vi "g2_2D.vi"() -> ()   [LabVIEW 2020]
uses:
  <vilib>/Math Plots/2D Math Plots/2D Error Bar/2D Error Bar XCtrl/2D Error Bar.xctl
  C:/Program Files/Dotfast Consulting/Timetag Explorer 2.26/ttInterface.dll
  Program Files/Dotfast Consulting/Timetag Explorer 2.26/ttInterface.dll
  <vilib>/Utility/file.llb/Write Delimited Spreadsheet (I64).vi
  <vilib>/Math Plots/2D Math Plots/2D Error Bar/2D Error Bar Datatype/Public/Plot Helper (Fixed).vi
  <vilib>/Math Plots/2D Math Plots/2D Error Bar/2D Error Bar Datatype/2D Error Bar Datatype.lvclass
  <vilib>/Analysis/NI_AALBase.lvlib
panel:
  out "Intensity Graph":dbl[][](graph)
  out "Numeric 2":i32
  out "Current Delay":dbl
  out "appended array":i32[](array[numeric])
  out "ABC":refnum<class "2D Plot Datatype.lvclass">[](xcontrol)
  out "Numeric":i32
  in  "Acq Time (s)":dbl=0.1 format="%#_13g"
  out "BC":refnum<class "2D Plot Datatype.lvclass">[](xcontrol)
  in  "# Steps":i32
  in  "stop":bool
  in  "fileName":string
  in  "Folder":path
  in  "CTW in ns":dbl
  out "GetTimeCounter":i32
  out "GetResolution":dbl
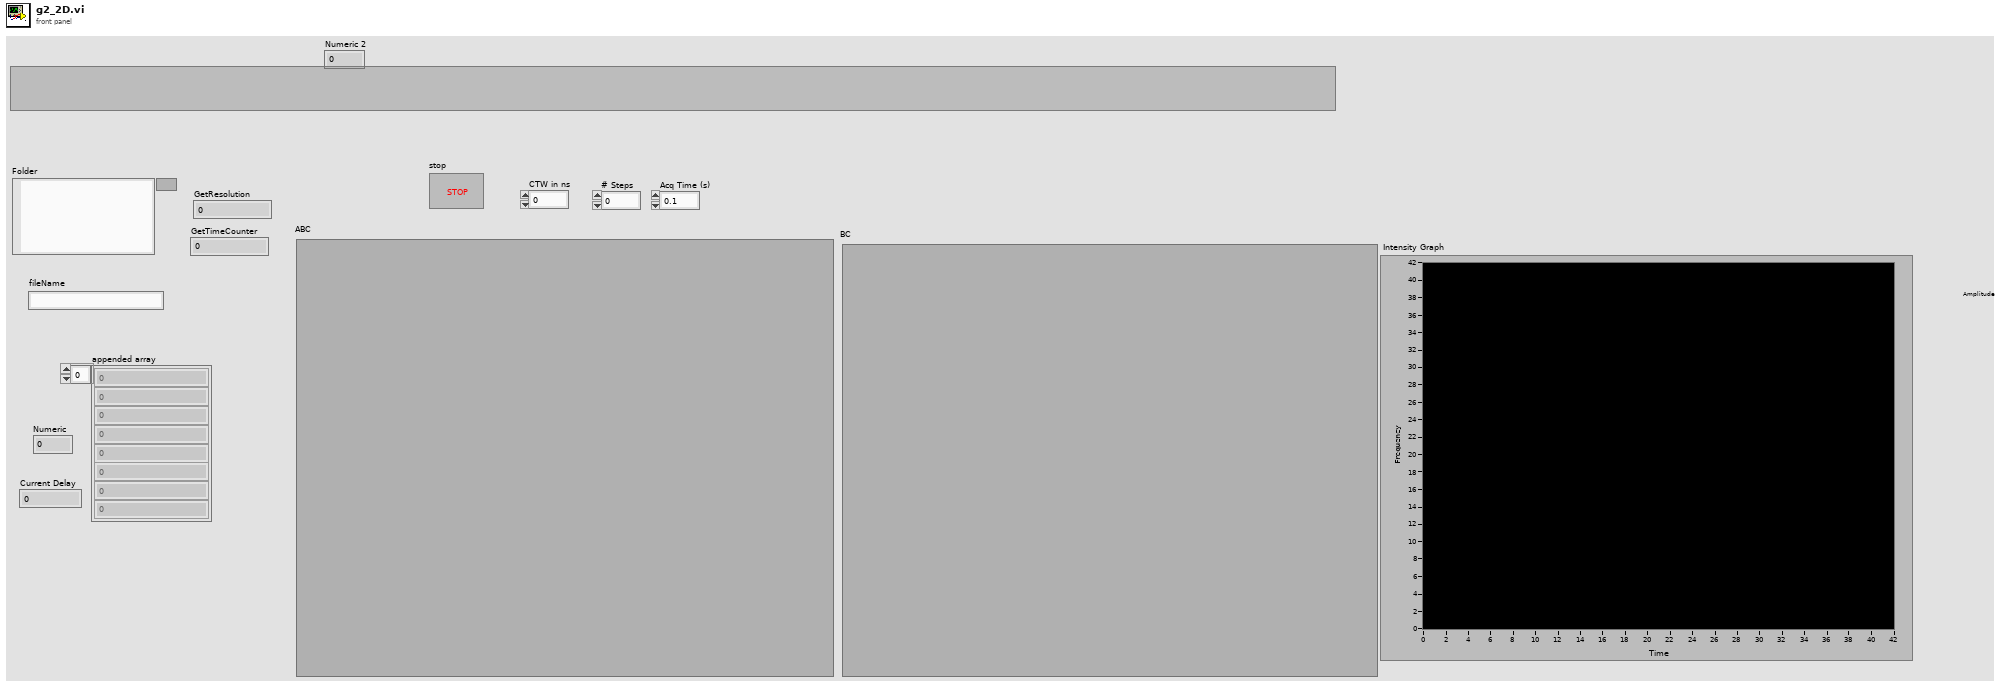
[diagram p1: front panel]
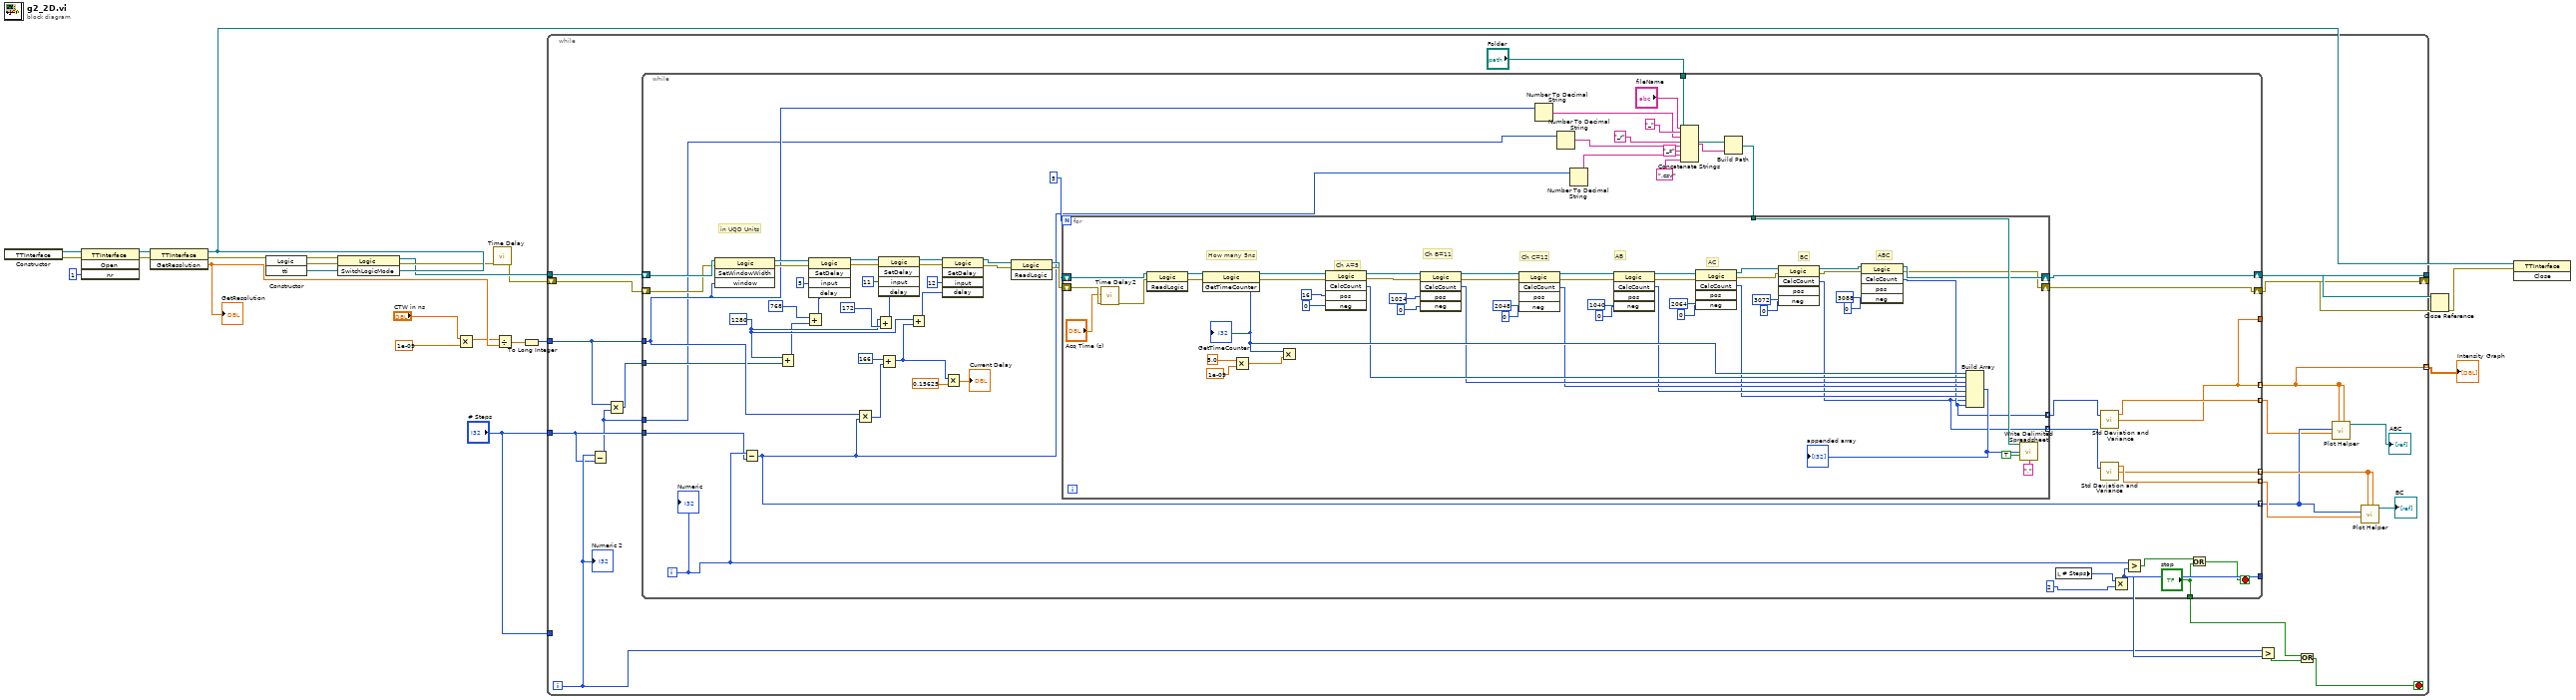
[diagram p0: block diagram]
diagram:
  n1 = constructor class="TTInterface"() -> (reference out=w23:refnum<k24>, error out=w22:errorcluster)  [unwired: 3 in, 1 out]
  n2 = invoke class="TTInterface" method="Open"(reference=w23, error in=w22, "nr"=1) -> (reference out=w19:refnum<k24>, error out=w20:errorcluster)  [unwired: 1 in, 2 out]
  n3 = invoke class="TTInterface" method="GetResolution"(reference=w19, error in=w20) -> (reference out=w18:refnum<k24>, error out=w17:errorcluster, "GetResolution"=w11:dbl)  [unwired: 1 in]
  "GetResolution" <- w11
  n4 = constructor class="Logic"(error in=w17, "tti"=w18) -> (reference out=w16:refnum<k24>, error out=w15:errorcluster)  [unwired: 2 in, 2 out]
  n5 = invoke class="Logic" method="SwitchLogicMode"(reference=w16, error in=w15) -> (reference out=w13:refnum<k24>, error out=w14:errorcluster)  [unwired: 1 in, 1 out]
  n6 = Multiply(x="CTW in ns", y=1e-09) -> (x*y=w10:dbl)
  n7 = call "Time Delay"("error in (no error)"=w14) -> ("error out"=w12:errorcluster)  [unwired: 10 in]
  n8 = Divide(x=w10, y=w11) -> (x/y=w9:dbl)
  n9 = To Long Integer(number=w9) -> (32bit integer=w6:i32)
  n10 = while {
    tunnel: w13 -> [w44]
    tunnel: w6 -> [w27]
    tunnel: "# Steps" -> [w28]
    shift-right: [w40] -> w3
    shift-left: w12 -> [w43]
    tunnel: [w41] -> w5
    tunnel: "# Steps" -> [_]
    tunnel: [w24] -> w1 mode=indexing
    i -> [w29]
    stop <- w30 stop-if-true
    n11 = Subtract(x=w29, y=w28) -> (x-y=w25:i32)
    n12 = Multiply(x=w27, y=w25) -> (x*y=w26:i32)
    n13 = while {
      shift-right: [w75] -> w41
      shift-left: w44 -> [w100]
      shift-right: [w74] -> w40
      shift-left: w43 -> [w99]
      tunnel: "Folder" -> [w94]
      tunnel: w27 -> [w81]
      tunnel: w28 -> [w78]
      tunnel: [w72] -> w34 mode=indexing
      tunnel: [w45] -> w24 mode=indexing
      tunnel: [w49] -> w35 mode=indexing
      tunnel: [w70] -> w36 mode=indexing
      tunnel: [w69] -> w37 mode=indexing
      tunnel: ["stop"] -> w33
      tunnel: [w53] -> w31
      tunnel: w26 -> [w47]
      tunnel: w25 -> [w46]
      tunnel: [w45] -> _
      i -> [w79]
      stop <- w91 stop-if-true
      w55 = 1280
      # "in UQD Units"
      n14 = invoke class="Logic" method="SetWindowWidth"(reference=w100, error in=w99, "window"=w81) -> (reference out=w98:refnum<k24>, error out=w97:errorcluster)  [unwired: 1 in, 2 out]
      n15 = Subtract(x=w79, y=w78) -> (x-y=w49:i32)
      n16 = Add(x=w55, y=w47) -> (x+y=w48:i32)
      n17 = Add(x=768 ("delay"), y=w48) -> (x+y=w59:i32)
      n18 = invoke class="Logic" method="SetDelay"(reference=w98, error in=w97, "input"=5, "delay"=w59) -> (reference out=w96:refnum<k24>, error out=w95:errorcluster)  [unwired: 1 in, 3 out]
      n19 = Multiply(x=w81, y=w49) -> (x*y=w80:i32)
      n20 = Add(x=w55, y=172 ("delay")) -> (x+y=w57:i32)
      n21 = invoke class="Logic" method="SetDelay"(reference=w96, error in=w95, "input"=11, "delay"=w57) -> (reference out=w89:refnum<k24>, error out=w88:errorcluster)  [unwired: 1 in, 3 out]
      n22 = Add(x=166 ("delay"), y=w80) -> (x+y=w62:i32)
      n23 = Add(x=w55, y=w62) -> (x+y=w56:i32)
      n24 = invoke class="Logic" method="SetDelay"(reference=w89, error in=w88, "input"=12, "delay"=w56) -> (reference out=w87:refnum<k24>, error out=w86:errorcluster)  [unwired: 1 in, 3 out]
      n25 = Multiply(x=w62, y=0.15625) -> (x*y=→"Current Delay":dbl)
      n26 = invoke class="Logic" method="ReadLogic"(reference=w87, error in=w86) -> (reference out=w102:refnum<k24>, error out=w103:errorcluster)  [unwired: 1 in, 1 out]
      n27 = Number To Decimal String(number=w81) -> (decimal integer string=w66:string)  [unwired: 1 in]
      n28 = Number To Decimal String(number=w46) -> (decimal integer string=w64:string)  [unwired: 1 in]
      n29 = Number To Decimal String(number=w49) -> (decimal integer string=w51:string)  [unwired: 1 in]
      n30 = Concatenate Strings("fileName", "_" ("string"), w66, "_r" ("string"), w64, "_s" ("string"), w51, ".csv" ("string")) -> (w92:string)
      n31 = Build Path(base path=w94, name or relative path=w92) -> (appended path=w93:path)
      n32 = for {
        N: 5 -> [_]
        shift-right: [w113] -> w74
        shift-left: w103 -> [w154]
        shift-right: [w114] -> w75
        shift-left: w102 -> [w153]
        tunnel: w93 -> [w140]
        tunnel: [w105] -> w73 mode=indexing
        tunnel: [w104] -> w71 mode=indexing
        # "ABC"
        # "BC"
        # "AC"
        # "AB"
        # "Ch C=12"
        # "Ch B=11"
        # "Ch A=5"
        # "How many 5ns"
        n33 = call "Time Delay2"("error in (no error)"=w154, "Delay Time (s)"="Acq Time (s)") -> ("error out"=w152:errorcluster)  [unwired: 9 in]
        n34 = invoke class="Logic" method="ReadLogic"(reference=w153, error in=w152) -> (reference out=w147:refnum<k24>, error out=w146:errorcluster)  [unwired: 1 in, 1 out]
        n35 = invoke class="Logic" method="GetTimeCounter"(reference=w147, error in=w146) -> (reference out=w144:refnum<k24>, error out=w143:errorcluster, "GetTimeCounter"=w112:i32)  [unwired: 1 in]
        "GetTimeCounter" <- w112
        n36 = Multiply(x=5.0, y=1e-09) -> (x*y=w148:dbl)
        n37 = Multiply(x=w112, y=w148) -> ()  [unwired: 1 out]
        n38 = invoke class="Logic" method="CalcCount"(reference=w144, error in=w143, "pos"=16, "neg"=0) -> (reference out=w136:refnum<k24>, error out=w135:errorcluster, "CalcCount"=w111:i32)  [unwired: 1 in, 2 out]
        n39 = invoke class="Logic" method="CalcCount"(reference=w136, error in=w135, "pos"=1024, "neg"=0) -> (reference out=w132:refnum<k24>, error out=w131:errorcluster, "CalcCount"=w110:i32)  [unwired: 1 in, 2 out]
        n40 = invoke class="Logic" method="CalcCount"(reference=w132, error in=w131, "pos"=2048, "neg"=0) -> (reference out=w128:refnum<k24>, error out=w127:errorcluster, "CalcCount"=w109:i32)  [unwired: 1 in, 2 out]
        n41 = invoke class="Logic" method="CalcCount"(reference=w128, error in=w127, "pos"=1040, "neg"=0) -> (reference out=w124:refnum<k24>, error out=w123:errorcluster, "CalcCount"=w108:i32)  [unwired: 1 in, 2 out]
        n42 = invoke class="Logic" method="CalcCount"(reference=w124, error in=w123, "pos"=2064, "neg"=0) -> (reference out=w119:refnum<k24>, error out=w120:errorcluster, "CalcCount"=w107:i32)  [unwired: 1 in, 2 out]
        n43 = invoke class="Logic" method="CalcCount"(reference=w119, error in=w120, "pos"=3072, "neg"=0) -> (reference out=w116:refnum<k24>, error out=w115:errorcluster, "CalcCount"=w104:i32)  [unwired: 1 in, 2 out]
        n44 = invoke class="Logic" method="CalcCount"(reference=w116, error in=w115, "pos"=3088, "neg"=0) -> (reference out=w114:refnum<k24>, error out=w113:errorcluster, "CalcCount"=w105:i32)  [unwired: 1 in, 2 out]
        n45 = Build Array(w112, w111, w110, w109, w108, w107, w104, w105) -> (w106:i32[])
        "appended array" <- w106
        n46 = call-poly <vilib>:"Write Delimited Spreadsheet.vi"("file path (dialog if empty)"=w140, "1D data"=w106, "append to file? (new file:F)"=TRUE, "delimiter (\\t)"="," ("delimiter (\\t)")) -> ()  [unwired: 10 in, 2 out]
      }
      n47 = local read "# Steps"() -> (w77:i32)
      n48 = call <vilib>:"Std Deviation and Variance.vi"("X"=w73) -> ("mean"=w72:dbl, "standard deviation"=w45:dbl)  [unwired: 1 in, 1 out]
      n49 = call <vilib>:"Std Deviation and Variance.vi"("X"=w71) -> ("mean"=w70:dbl, "standard deviation"=w69:dbl)  [unwired: 1 in, 1 out]
      n50 = Multiply(x=w77, y=2) -> (x*y=w53:i32)
      n51 = Greater?(x=w79, y=w53) -> (0:w90:bool)
      n52 = Or(x=w90, y="stop") -> (x .or. y?=w91:bool)
      "Numeric" <- w79
    }
    n53 = Greater?(x=w29, y=w31) -> (0:w32:bool)
    n54 = Or(x=w33, y=w32) -> (x .or. y?=w30:bool)
    n55 = call-poly <vilib>:"Plot Helper.vi"("error b vector"=w24, "error a vector"=w24, "y vector"=w34, "x vector"=w35) -> ("2D Plot Class Obj Array out"=→"ABC":refnum<class "2D Plot Datatype.lvclass">[])  [unwired: 2 in, 5 out]
    n56 = call-poly <vilib>:"Plot Helper.vi"("error b vector"=w37, "error a vector"=w37, "y vector"=w36, "x vector"=w35) -> ("2D Plot Class Obj Array out"=→"BC":refnum<class "2D Plot Datatype.lvclass">[])  [unwired: 2 in, 5 out]
    "Numeric 2" <- w29
  }
  "Intensity Graph" <- w1
  n57 = Close Reference(reference=w5, error in (no error)=w3) -> (error out=w4:errorcluster)
  n58 = invoke class="TTInterface" method="Close"(reference=w18, error in=w4) -> ()  [unwired: 1 in, 3 out]
